vi "Set End Point.vi"(8 "error in (no error)":errorcluster, 10 "end point (0,0)":cluster{"x":i16, "y":i16}, 11 "Graphics Object.lvclass in":refnum<class "Graphics Object.lvclass">) -> (0 "error out":errorcluster, 3 "Graphics Object.lvclass out":refnum<class "Graphics Object.lvclass">)   [LabVIEW 2020, in "Graphics Object.lvclass"]
doc: "Set the end point of a bounding box surrounding a graphics object"
uses:
  Graphics Object.lvclass
  Graphics Object.lvclass/Graphics Object.ctl
panel:
  # "expressionflow.com"
  # "Copyright (c) 2008 Tomi Maila. All rights reserved."
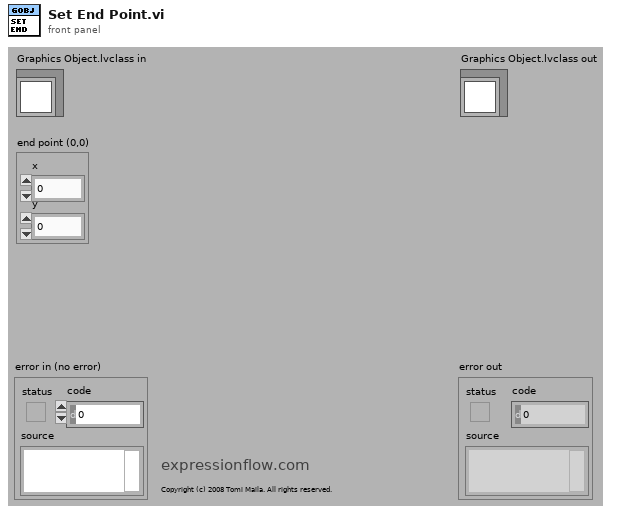
[diagram p1: front panel]
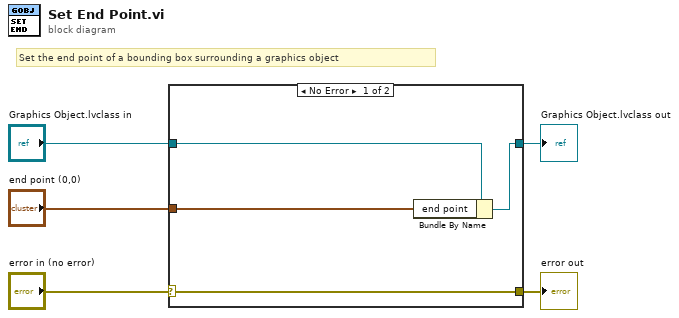
[diagram p0: block diagram]
diagram:
  # "Set the end point of a bounding box surrounding a graphics object"
  n1 = case shown="No Error" "error in (no error)" {
    selector: "error in (no error)" -> [w9 w10]
    tunnel: [w9 w10] -> w4
    tunnel: [w7 w11] -> w2
    tunnel: "Graphics Object.lvclass in" -> [w8 w11]
    tunnel: "end point (0,0)" -> [w6 _]
    frame No Error {
      n2 = Bundle By Name(cluster=w8, "end point"=w6) -> (w7:refnum<class "Graphics Object.lvclass">)
    }
    frame Error {
    }
  }
  "error out" <- w4
  "Graphics Object.lvclass out" <- w2
